vi "CAL_GCP_L_fpga.vi"(10 "IMU_init_L":sgl, 11 "L_ROLL":sgl) -> (0 "L_Period":i16, 1 "L_GCP":sgl, 3 "L_NUM":u32)   [LabVIEW 2019]
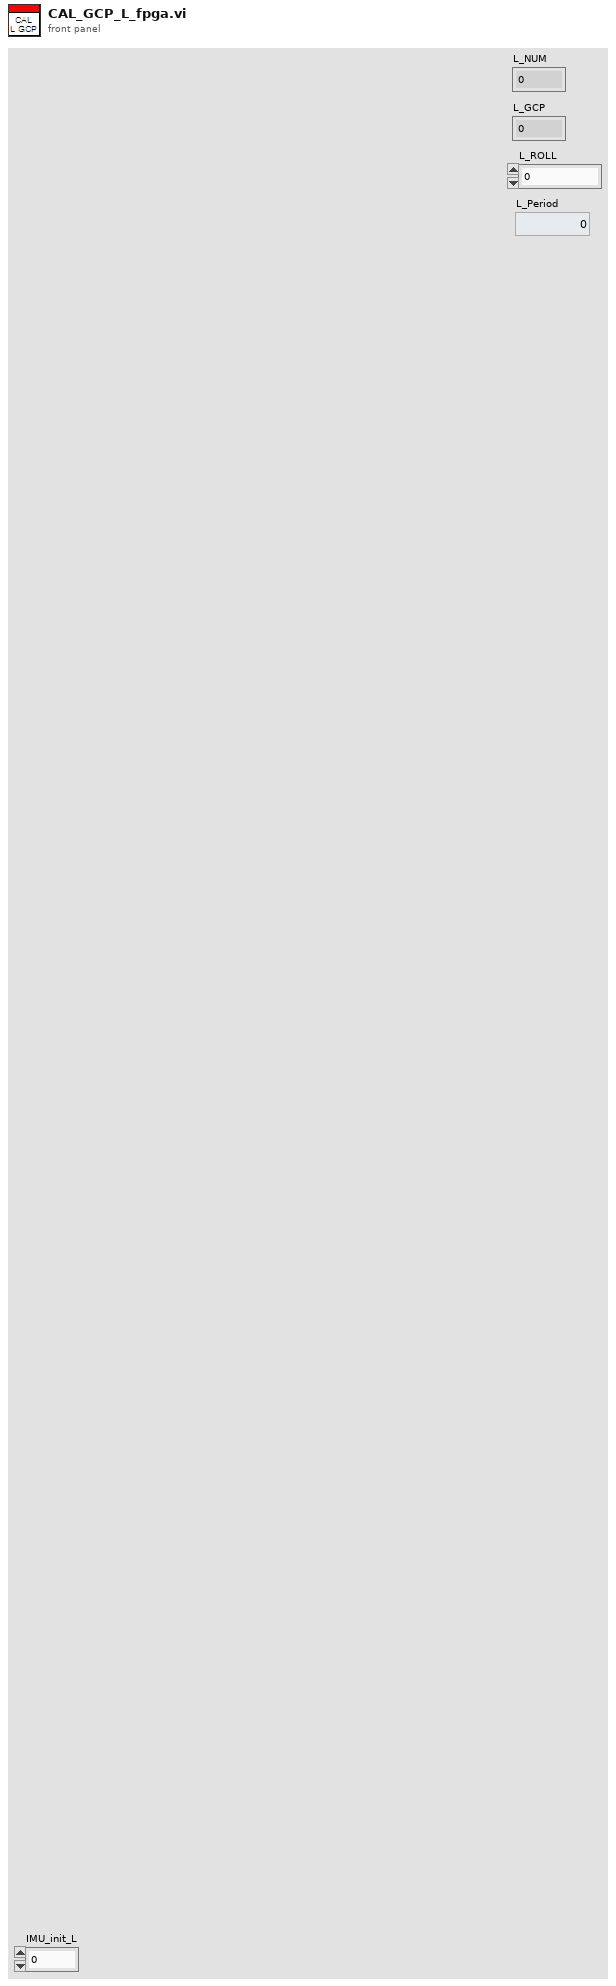
[diagram p1: front panel]
types:
  T1 = enum16{"Init", "HF", "Cross", "HE", "Cross_E", "Init_F"}
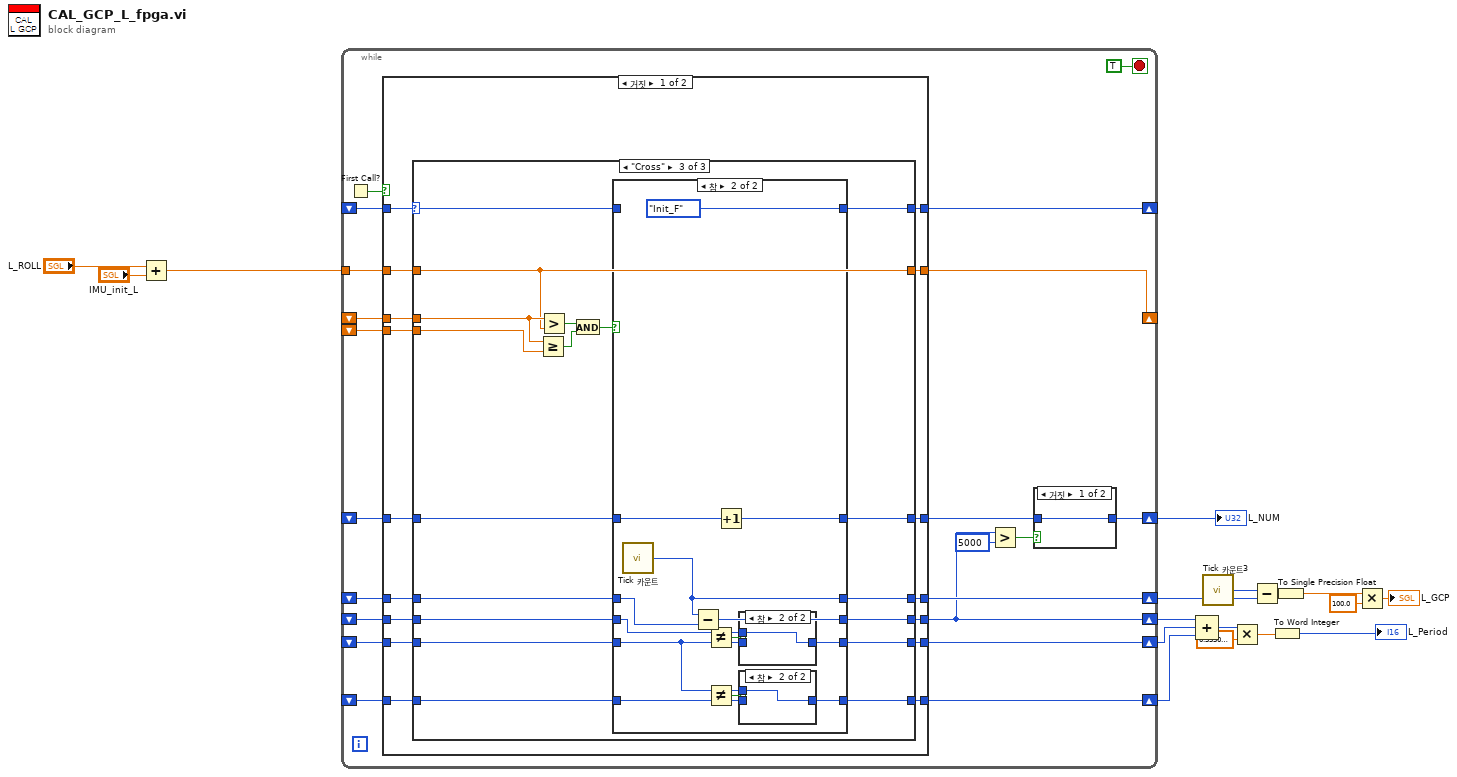
[diagram p0: block diagram]
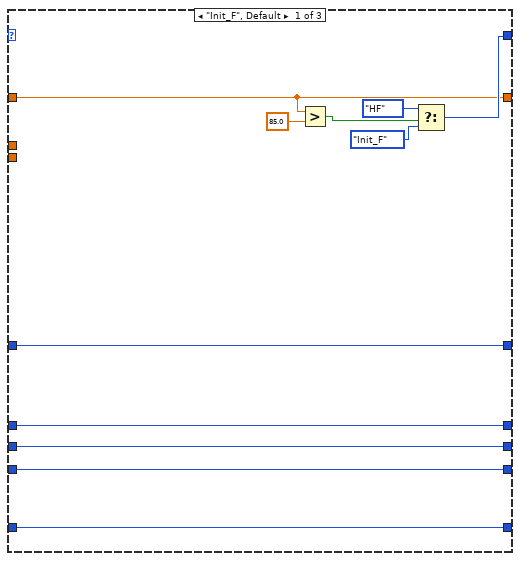
[diagram p2: hidden frame]
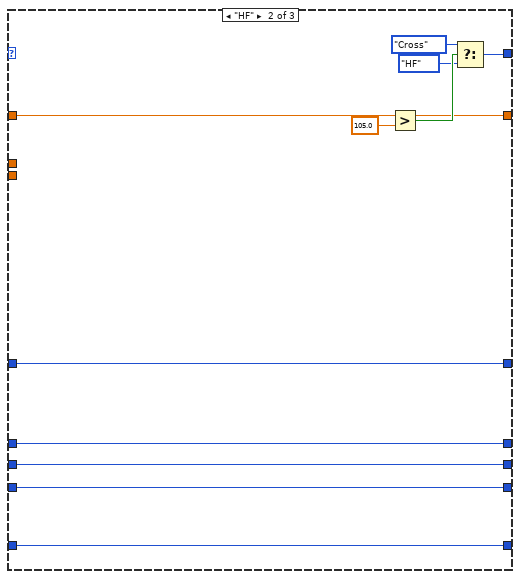
[diagram p3: hidden frame]
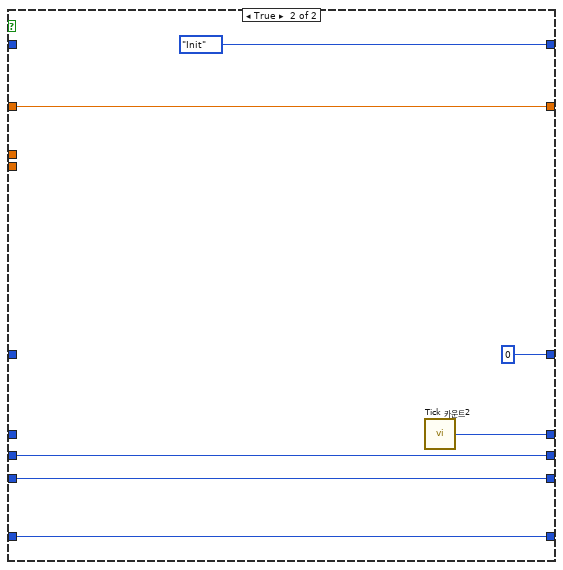
[diagram p7: hidden frame]
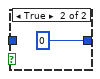
[diagram p8: hidden frame]
diagram:
  n1 = Add(x="L_ROLL", y="IMU_init_L") -> (x+y=w11:sgl)
  n2 = while {
    tunnel: w11 -> [w35]
    shift-right: [w20] -> _
    shift-left: _ -> [w19]
    shift-right: [w36] -> _
    shift-left: _ -> [w33]
    shift-left: _ -> [w32]
    shift-right: [w29] -> w14
    shift-left: _ -> [w34]
    shift-right: [w25] -> w7
    shift-left: _ -> [w24]
    shift-right: [w22] -> w6
    shift-left: _ -> [w23]
    shift-right: [w27] -> w13
    shift-left: _ -> [w26]
    shift-right: [w18] -> w8
    shift-left: _ -> [w21]
    stop <- TRUE stop-if-true
    n3 = First Call?() -> (First Call?: T/F=w37:bool)
    n4 = case shown="거짓" w37 {
      tunnel: [w53 w124] -> w36
      tunnel: w35 -> [w54 w124]
      tunnel: w34 -> [w51 _]
      tunnel: [w52 u32 0] -> w28
      tunnel: w33 -> [w50 _]
      tunnel: w32 -> [w49 _]
      tunnel: [w48 w118] -> w27
      tunnel: w26 -> [w47 _]
      tunnel: [w46 w122] -> w25
      tunnel: w24 -> [w45 w122]
      tunnel: w23 -> [w44 w121]
      tunnel: [w43 w121] -> w22
      tunnel: [w42 w120] -> w18
      tunnel: w21 -> [w41 w120]
      tunnel: [w39 T1."Init"] -> w20
      tunnel: w19 -> [w40 _]
      frame False {
        n5 = case shown="\"Cross\"" w40 {
          selector: w40 -> [_ _ w94]
          tunnel: w54 -> [w62 w75 w87]
          tunnel: [w62 w75 w87] -> w53
          tunnel: [w61 w74 w89] -> w52
          tunnel: w51 -> [w61 w74 w90]
          tunnel: w50 -> [_ _ w88]
          tunnel: w49 -> [_ _ w93]
          tunnel: [w60 w73 w85] -> w48
          tunnel: w47 -> [w60 w73 w84]
          tunnel: [w58 w72 w83] -> w46
          tunnel: w45 -> [w58 w72 w82]
          tunnel: w44 -> [w57 w71 w81]
          tunnel: [w57 w71 w80] -> w43
          tunnel: [w59 w70 w79] -> w42
          tunnel: w41 -> [w59 w70 w78]
          tunnel: [w63 w67 w77] -> w39
          frame "Init_F", Default {
            n6 = Greater?(x=w62, y=sgl 85.0) -> (0:w56:bool)
            n7 = Select(t=T1."HF", s=w56, f=T1."Init_F") -> (s? t:f=w63:T1)
          }
          frame "HF" {
            n8 = Greater?(x=w75, y=sgl 105.0) -> (0:w76:bool)
            n9 = Select(t=T1."Cross", s=w76, f=T1."HF") -> (s? t:f=w67:T1)
          }
          frame "Cross" {
            n10 = Greater Or Equal?(x=w88, y=w93) -> (x >= y?=w92:bool)
            n11 = Greater?(x=w88, y=w87) -> (0:w86:bool)
            n12 = And(x=w86, y=w92) -> (x .and. y?=w91:bool)
            n13 = case shown="참" w91 {
              tunnel: w94 -> [w99 _]
              tunnel: [w99 T1."Init_F"] -> w77
              tunnel: w90 -> [w100 w105]
              tunnel: [w100 w104] -> w89
              tunnel: [w98 w101] -> w85
              tunnel: w84 -> [w98 w111]
              tunnel: [w97 w110] -> w83
              tunnel: w82 -> [w97 w102]
              tunnel: w81 -> [w96 w109]
              tunnel: [w96 w108] -> w80
              tunnel: [w95 w107] -> w79
              tunnel: w78 -> [w95 w103]
              frame False {
              }
              frame True {
                n14 = call "Tick 카운트"() -> ("Tick Count(mSec)"=w101:u32)
                n15 = Subtract(x=w101, y=w111) -> (x-y=w107:u32)
                n16 = Not Equal?(x=w103, y=w102) -> (x != y?=w113:bool)
                n17 = Not Equal?(x=w102, y=w109) -> (x != y?=w112:bool)
                n18 = Increment(x=w105) -> (x+1=w104:u32)
                n19 = case shown="참" w113 {
                  tunnel: w103 -> [_ w117]
                  tunnel: [w116 w117] -> w110
                  tunnel: w102 -> [w116 _]
                  frame False {
                  }
                  frame True {
                  }
                }
                n20 = case shown="참" w112 {
                  tunnel: w102 -> [_ w115]
                  tunnel: w109 -> [w114 _]
                  tunnel: [w114 w115] -> w108
                  frame False {
                  }
                  frame True {
                  }
                }
              }
            }
          }
        }
      }
      frame True {
        n21 = call "Tick 카운트2"() -> ("Tick Count(mSec)"=w118:u32)
      }
    }
    n22 = Greater?(x=w18, y=u32 5000) -> (0:w30:bool)
    n23 = case shown="거짓" w30 {
      tunnel: [w125 u32 0] -> w29
      tunnel: w28 -> [w125 _]
      frame False {
      }
      frame True {
      }
    }
  }
  "L_NUM" <- w14
  n24 = Compound Arithmetic op=ADD(w8, w7, w6) -> (w3:u32)
  n25 = call "Tick 카운트3"() -> ("Tick Count(mSec)"=w10:u32)
  n26 = Multiply(x=w3, y=sgl 0.333) -> (x*y=w1:sgl)
  n27 = Subtract(x=w10, y=w13) -> (x-y=w16:u32)
  n28 = To Word Integer(number=w1) -> (16bit integer=→"L_Period":i16)
  n29 = To Single Precision Float(number=w16) -> (single precision float=w5:sgl)
  n30 = Multiply(x=w5, y=sgl 100.0) -> (x*y=→"L_GCP":sgl)
